vi "SetParent.vi"(8 "error in":errorcluster, 9 "hWndNewParent":u32, 10 "hWndChild":i32) -> (0 "error out":errorcluster, 1 "hWndNewParent Out":u32, 2 "hWndChild Out":i32, 3 "Returned hWnd":u32)   [LabVIEW 2009]
uses:
  user32.dll
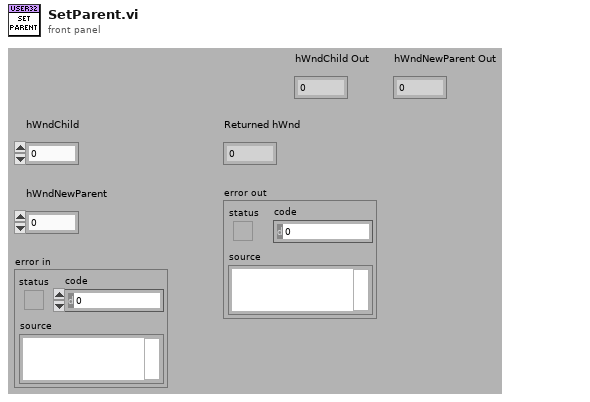
[diagram p1: front panel]
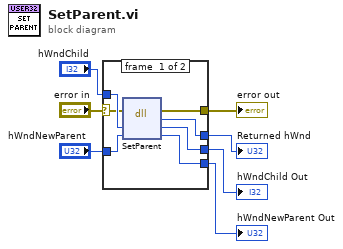
[diagram p0: block diagram]
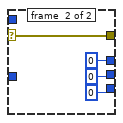
[diagram p2: hidden frame]
diagram:
  n1 = case shown="No Error" "error in" {
    selector: "error in" -> [w10 w18]
    tunnel: "hWndNewParent" -> [w14 _]
    tunnel: "hWndChild" -> [w13 _]
    tunnel: [w12 u32 0 ("hWnd")] -> w5
    tunnel: [w11 w18] -> w4
    tunnel: [w9 0 ("hWndChild")] -> w2
    tunnel: [w8 u32 0 ("hWndNewParent")] -> w1
    frame #0 {
      n2 = dll-call lib="user32.dll" fn="SetParent"(error in=w10, "hWndChild"=w13, "hWndNewParent"=w14) -> (error out=w11:errorcluster, "hWnd"=w12:u32, "hWndChild"=w9:i32, "hWndNewParent"=w8:u32)  [unwired: 2 in, 1 out]
    }
    frame #1 {
    }
  }
  "Returned hWnd" <- w5
  "error out" <- w4
  "hWndChild Out" <- w2
  "hWndNewParent Out" <- w1
